vi "Target Initiate Communication Queues.vi"(8 "Error In":errorcluster) -> (0 "Refnum out":refnum<k33>, 1 "Error Out":errorcluster, 3 "writer name":refnum<k21>)   [LabVIEW 2018]
uses:
  Target Logging Cluster.ctl
  Target Sensors.ctl
  Host Messages.ctl
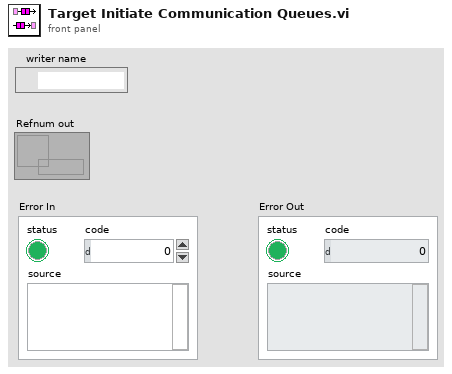
[diagram p1: front panel]
types:
  T1 = typedef "Host Messages.ctl" = enum16{"Stop", "Log Data", "Confirm File Name"}
  T2 = typedef "Target Logging Cluster.ctl" = cluster{"Valid for Logging?":bool, "Target Sensors":T3}
  T3 = typedef "Target Sensors.ctl" = cluster{"Raw Cable Force (N)":dbl, "Prosthesis Angle (deg)":dbl, "Main Clock Line (s)":dbl}
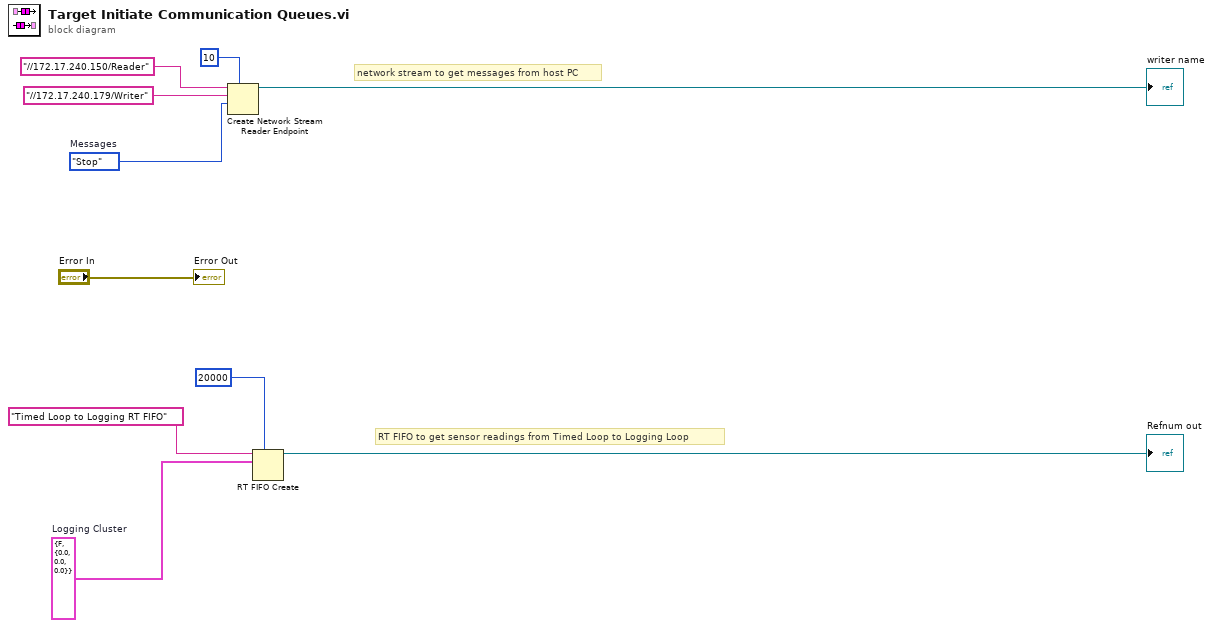
[diagram p0: block diagram]
diagram:
  w1 = Host_Messages."Stop"  # Messages
  w10 = T2 {"Valid for Logging?"=FALSE, "Target Sensors"={"Raw Cable Force (N)"=0.0, "Prosthesis Angle (deg)"=0.0, "Main Clock Line (s)"=0.0}}  # Logging Cluster
  # "RT FIFO to get sensor readings from Timed Loop to Logging Loop"
  # "network stream to get messages from host PC"
  n1 = Create Network Stream Reader Endpoint(7:10 ("reader buffer size"), 9:w1, 10:"//172.17.240.179/Writer" ("writer name"), 11:"//172.17.240.150/Reader" ("writer name")) -> (3:→"writer name":refnum<k21>)  [unwired: 3 in, 1 out]
  n2 = RT FIFO Create(0:"Timed Loop to Logging RT FIFO" ("name (unnamed)"), 1:w10, 4:u32 20000 ("size (10)")) -> (8:→"Refnum out":refnum<k33>)  [unwired: 5 in, 2 out]
  "Error Out" <- "Error In"
